vi "lvstyx_log_message.vi"(6 "File Length":i32, 7 "Logging Enable (T)":bool=TRUE, 8 "error in (no error)":errorcluster, 9 "Read? (F)":bool, 10 "File value":string, 11 "File Name":string) -> (4 "error out":errorcluster)   [LabVIEW 2010, in "lib1299.lvlib"]
doc: "This VI creates and displays a message to the user showing the estyx file, value, and sucess of the read/write function called.\n\nInputs:\nFile Name - estyx filename the operation relates to\nFile Value - value read/written to the estyx file\nFile Length - length of the estyx file\nRead - Read or Write operation (default: F = write)\nLogging Enable - Enable messaging to user (default: F = no messages displayed)\nerror in - error input cluster\n\nOutputs:\nError out - error output cluster\n\nOutputs:"
uses:
  lib1299.lvlib
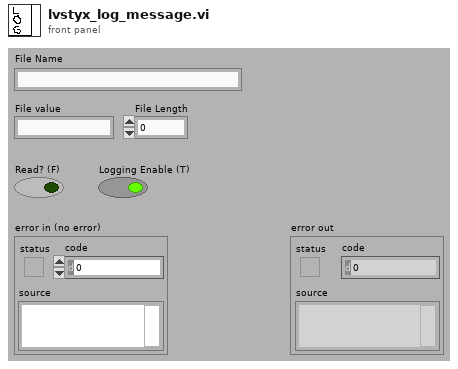
[diagram p1: front panel]
types:
  T1 = enum16{"open", "replace", "create", "open or create", "replace or create", "replace or create with confirmation"}
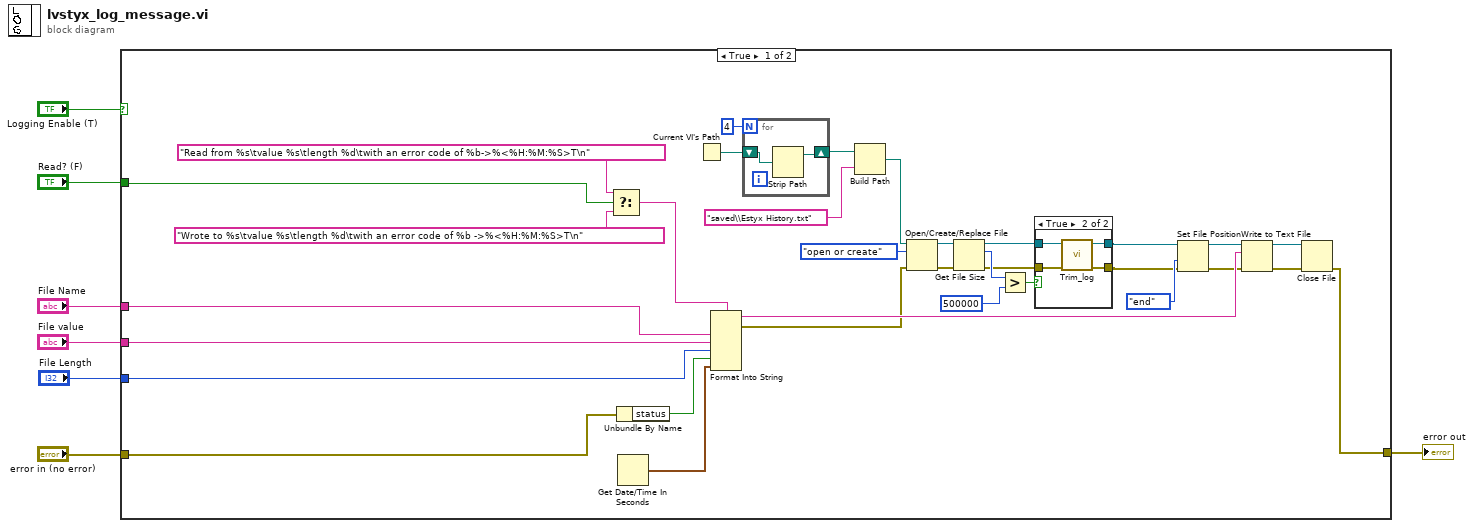
[diagram p0: block diagram]
diagram:
  n1 = case shown="True" "Logging Enable (T)" {
    tunnel: "File Name" -> [w40 _]
    tunnel: "error in (no error)" -> [w27 w49]
    tunnel: "File value" -> [w39 _]
    tunnel: "Read? (F)" -> [w36 _]
    tunnel: [w26 w49] -> w3
    tunnel: "File Length" -> [w34 _]
    frame True {
      n2 = Select(t="Read from %s\tvalue %s\tlength %d\twith an error code of %b->%<%H:%M:%S>T\n" ("format string"), s=w36, f="Wrote to %s\tvalue %s\tlength %d\twith an error code of %b ->%<%H:%M:%S>T\n" ("format string")) -> (s? t:f=w38:string)
      n3 = Unbundle By Name(w27) -> ("status"=w33:bool)
      n4 = Get Date/Time In Seconds() -> (seconds since 1Jan1904=w25:timestamp)
      n5 = Current VI's Path() -> (path=w32:path)
      n6 = Format Into String(format string=w38, w40, w39, w34, w33, w25) -> (resulting string=w28:string, error out=w13:errorcluster)  [unwired: 2 in]
      n7 = for {
        N: 4 -> [_]
        shift-right: [w47] -> w30
        shift-left: w32 -> [w48]
        n8 = Strip Path(path=w48) -> (stripped path=w47:path)  [unwired: 1 out]
      }
      n9 = Build Path(base path=w30, name or relative path="saved\\Estyx History.txt") -> (appended path=w15:path)
      n10 = Open/Create/Replace File(file path (use dialog)=w15, error in=w13, operation (0:open)=T1."open or create") -> (refnum out=w21:refnum<file>, error out=w12:errorcluster)  [unwired: 3 in, 1 out]
      n11 = Get File Size(file=w21, error in=w12) -> (refnum out=w10:refnum<file>, size (in bytes)=w24:i64, 0:w11:errorcluster)
      n12 = Greater?(x=w24, y=i64 500000) -> (0:w14:bool)
      n13 = case shown="True" w14 {
        tunnel: w11 -> [w41 w46]
        tunnel: w10 -> [w42 w45]
        tunnel: [w41 w44] -> w8
        tunnel: [w42 w43] -> w9
        frame False {
        }
        frame True {
          n14 = call "Trim_log.vi"("error in (no error)"=w46, "Log File Refnum"=w45) -> ("error out"=w44:errorcluster, "Log File Refnum (out)"=w43:refnum<file>)  [unwired: 8 in]
        }
      }
      n15 = Set File Position(refnum=w9, from (0:start)=enum16{"start", "end", "current"}."end", error in=w8) -> (refnum out=w18:refnum<file>, error out=w19:errorcluster)  [unwired: 1 in]
      n16 = Write to Text File(file (use dialog)=w18, text=w28, error in=w19) -> (refnum out=w16:refnum<file>, error out=w17:errorcluster)  [unwired: 1 in, 1 out]
      n17 = Close File(refnum=w16, error in=w17) -> (error out=w26:errorcluster)  [unwired: 1 out]
    }
    frame False {
    }
  }
  "error out" <- w3
